vi "GetLines.vi"(9 "delimiter":string="\n", 11 "String":string) -> (3 "Array":string[](array[string]))   [LabVIEW 2022 SP3]
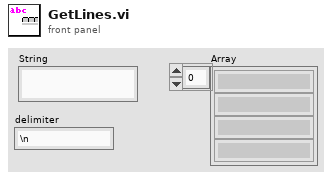
[diagram p1: front panel]
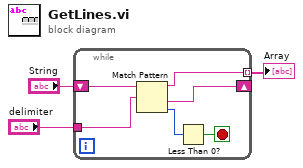
[diagram p0: block diagram]
diagram:
  n1 = while {
    shift-right: [w8] -> _
    shift-left: "String" -> [w9]
    tunnel: [w7] -> w1 mode=indexing
    tunnel: "delimiter" -> [w4]
    stop <- w5 stop-if-true
    n2 = Match Pattern(string=w9, regular expression=w4) -> (before substring=w7:string, after substring=w8:string, offset past match=w6:i32)  [unwired: 1 in, 1 out]
    n3 = Less Than 0?(x=w6) -> (x < 0?=w5:bool)
  }
  "Array" <- w1
